vi "Device Erase.vi"(8 "error in (no error)":errorcluster, 9 "End Sector":u8, 10 "Start Sector":u8, 11 "Option":enum16{"Erase Full Chip", "Erase Sectors"}(ring)) -> (0 "error out":errorcluster, 3 "Erase OK?":bool)   [LabVIEW 2015, in "ST-Link.lvlib"]
doc: "芯片擦除。\nOptions: Earase Full Chip --> 擦除整个芯片；Erase Sectors --> 擦除指定扇区；\nStart Sector: 指定起始扇区号，仅在选择Erase Sectors时才需要指定；\nEnd Sector: 指定结束扇区号，仅在选择Erase Sectors时才需要指定；\n\n[Erase OK?]: 返回擦除状态；"
uses:
  ST-Link.lvlib
  <vilib>/regexp/Match Regular Expression.xnode
panel:
  out "standard output":string
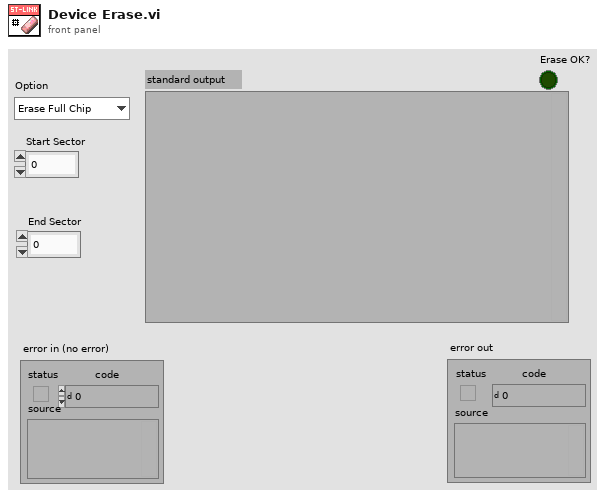
[diagram p1: front panel]
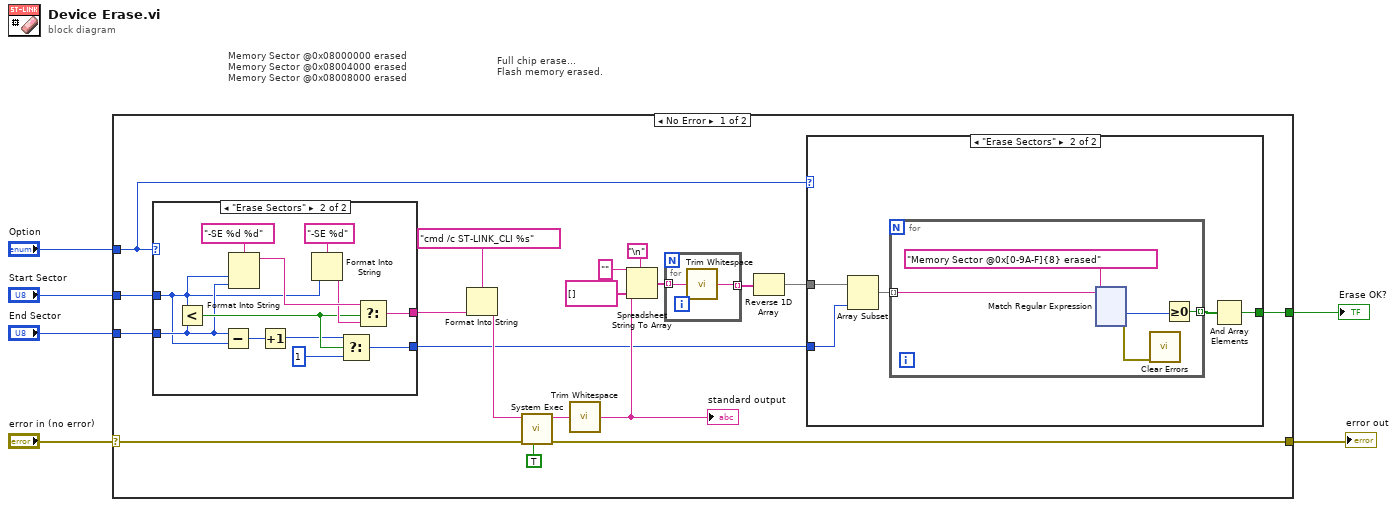
[diagram p0: block diagram]
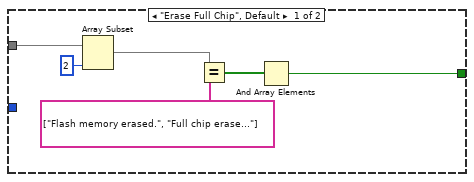
[diagram p2: hidden frame]
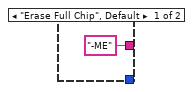
[diagram p3: hidden frame]
diagram:
  # "Full chip erase...\nFlash memory erased."
  # "Memory Sector @0x08000000 erased\nMemory Sector @0x08004000 erased\nMemory Sector @0x08008000 erased"
  n1 = case shown="No Error" "error in (no error)" {
    selector: "error in (no error)" -> [w24 w171]
    tunnel: [w23 w171] -> w5
    tunnel: "Option" -> [w10 _]
    tunnel: "Start Sector" -> [w15 _]
    tunnel: "End Sector" -> [w14 _]
    tunnel: [w7 _] -> w1
    frame No Error {
      n2 = case shown="\"Erase Sectors\"" w10 {
        tunnel: w15 -> [_ w161]
        tunnel: w14 -> [_ w162]
        tunnel: ["-ME" w164] -> w12
        tunnel: [_ w157] -> w9
        frame "Erase Full Chip", Default {
        }
        frame "Erase Sectors" {
          n3 = Less?(x=w161, y=w162) -> (x < y?=w163:bool)
          n4 = Subtract(x=w162, y=w161) -> (x-y=w160:u8)
          n5 = Format Into String(format string="-SE %d %d", w161, w162) -> (resulting string=w166:string)  [unwired: 2 in, 1 out]
          n6 = Increment(x=w160) -> (x+1=w159:u8)
          n7 = Format Into String(format string="-SE %d", w161) -> (resulting string=w165:string)  [unwired: 2 in, 1 out]
          n8 = Select(t=w159, s=w163, f=u8 1) -> (s? t:f=w157:u8)
          n9 = Select(t=w166, s=w163, f=w165) -> (s? t:f=w164:string)
        }
      }
      n10 = Format Into String(format string="cmd /c ST-LINK_CLI %s" ("command line"), w12) -> (resulting string=w11:string)  [unwired: 2 in, 1 out]
      n11 = call <vilib>:"System Exec.vi"("run minimized? (F)"=TRUE, "error in (no error)"=w24, "command line"=w11) -> ("error out"=w23:errorcluster, "standard output"=w22:string)  [unwired: 5 in, 2 out]
      n12 = call <vilib>:"Trim Whitespace.vi"("string"=w22) -> ("trimmed string"=w16:string)  [unwired: 1 in]
      "standard output" <- w16
      n13 = Spreadsheet String To Array(delimiter (Tab)="\n", format string="", spreadsheet string=w16, array type (2D Dbl)=string[] []) -> (array=w18:string[])
      n14 = for {
        tunnel: w18 -> [w170] mode=indexing
        tunnel: [w169] -> w17 mode=indexing
        n15 = call <vilib>:"Trim Whitespace.vi"("string"=w170) -> ("trimmed string"=w169:string)  [unwired: 1 in]
      }
      n16 = Reverse 1D Array(array=w17) -> (reversed array=w8:string[])
      n17 = case shown="\"Erase Sectors\"" w10 {
        tunnel: w9 -> [_ w35]
        tunnel: w8 -> [w31 w36]
        tunnel: [w26 w32] -> w7
        frame "Erase Full Chip", Default {
          n18 = Array Subset(array=w31, length=2) -> (w29:string[])  [unwired: 1 in]
          n19 = Equal?(x=w29, y=string[] ["Flash memory erased.", "Full chip erase..."]) -> (x = y?=w27:bool[])
          n20 = And Array Elements(Boolean array=w27) -> (logical AND=w26:bool)
        }
        frame "Erase Sectors" {
          n21 = Array Subset(array=w36, length=w35) -> (w34:string[])  [unwired: 1 in]
          n22 = for {
            tunnel: w34 -> [w41] mode=indexing
            tunnel: [w38] -> w33 mode=indexing
            n23 = xnode "Match Regular Expression"("input string"=w41, "regular expression"="Memory Sector @0x[0-9A-F]{8} erased") -> ("offset past match"=w39:i32, "error out"=w37:errorcluster)  [unwired: 4 in, 3 out]
            n24 = call <vilib>:"Clear Errors.vi"("error in (no error)"=w37) -> ()  [unwired: 5 in, 2 out]
            n25 = Greater Or Equal To 0?(x=w39) -> (x >= 0?=w38:bool)
          }
          n26 = And Array Elements(Boolean array=w33) -> (logical AND=w32:bool)
        }
      }
    }
    frame Error {
    }
  }
  "error out" <- w5
  "Erase OK?" <- w1
